vi "Get MAX rel move.vi"(0 "Zaber":T1={"Serial port handle"="", "Axis"="", "Controller #"=0, "Min position"=0.0, "Max position"=0.0, "Min velocity"=0.0, "Max velocity"=0.0, "Firmware"="", "Device ID"=0, "Variable event"=refnum, "Variable ref"=refnum, "Resolution, usteps/step"=0, "Serial port semaphore"=refnum, "Joystick buttons"={"MinDir"=1, "MaxDir"=2, "MedSpeed"=5, "HighSpeed"=6}} {"Joystick buttons"."HighSpeed" min=1 max=25 step=1; "Joystick buttons"."MedSpeed" min=1 max=25 step=1; "Joystick buttons"."MaxDir" min=1 max=25 step=1; "Joystick buttons"."MinDir" min=1 max=25 step=1}, 5 "error in":errorcluster) -> (14 "Zaber out":T1={"Serial port handle"="", "Axis"="", "Controller #"=0, "Min position"=0.0, "Max position"=0.0, "Min velocity"=0.0, "Max velocity"=0.0, "Firmware"="", "Device ID"=0, "Variable event"=refnum, "Variable ref"=refnum, "Resolution, usteps/step"=0, "Serial port semaphore"=refnum, "Joystick buttons"={"MinDir"=1, "MaxDir"=2, "MedSpeed"=5, "HighSpeed"=6}} {"Joystick buttons"."HighSpeed" min=1 max=25 step=1; "Joystick buttons"."MedSpeed" min=1 max=25 step=1; "Joystick buttons"."MaxDir" min=1 max=25 step=1; "Joystick buttons"."MinDir" min=1 max=25 step=1}, 16 "MAX rel move, usteps":i32, 19 "error out":errorcluster)   [LabVIEW 2017]
uses:
  CommandZaber.ctl
  GenericDataEvent/GenericEvent.ctl
  Zaber.ctl
  ZaberVariables.ctl
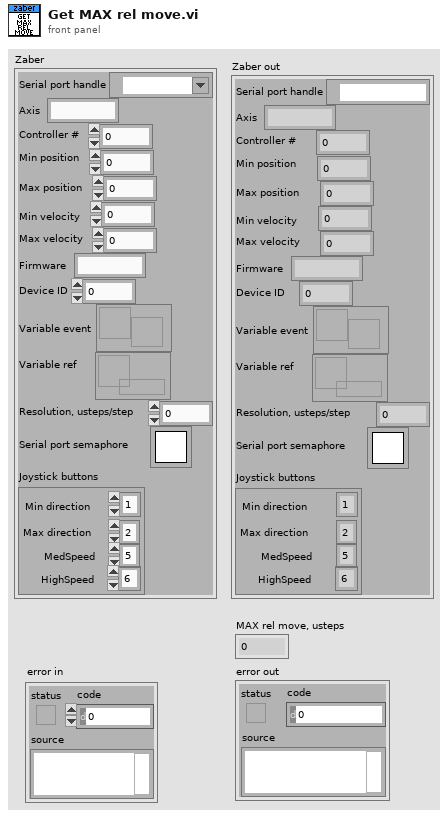
[diagram p1: front panel]
types:
  T1 = typedef "Zaber.ctl" = cluster{"Serial port handle":refnum<visa-resource-name>, "Axis":string, "Controller #":u8, "Min position":dbl, "Max position":dbl, "Min velocity":dbl, "Max velocity":dbl, "Firmware":string, "Device ID":i32, "Variable event":T2, "Variable ref":refnum<data-value>, "Resolution, usteps/step":i32, "Serial port semaphore":T3, "Joystick buttons":cluster{"MinDir":i32, "MaxDir":i32, "MedSpeed":i32, "HighSpeed":i32}}
  T2 = typedef "GenericEvent.ctl" = refnum<user-event>
  T3 = typedef "Semaphore RefNum" = refnum<k1>
  T4 = typedef "CommandZaber.ctl" = cluster{"Command":u8, "Data":i32}
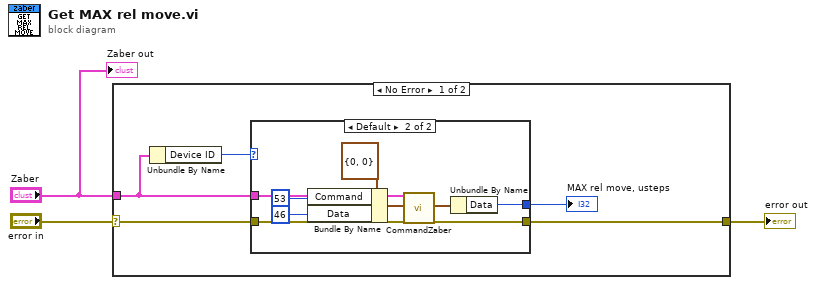
[diagram p0: block diagram]
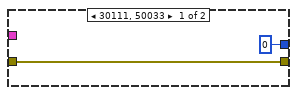
[diagram p2: hidden frame]
diagram:
  n1 = case shown="No Error" "error in" {
    selector: "error in" -> [w7 w20]
    tunnel: [w6 w20] -> w2
    tunnel: "Zaber" -> [w5 _]
    frame No Error {
      n2 = Unbundle By Name(w5) -> ("Device ID"=w4:i32)
      n3 = case shown="Default" w4 {
        tunnel: [0 ("Data") w19] -> w8
        tunnel: w7 -> [w10 w14]
        tunnel: [w10 w13] -> w6
        tunnel: w5 -> [_ w11]
        frame 30111, 50033 {
        }
        frame Default {
          n4 = Bundle By Name(cluster=T4 {"Command"=0, "Data"=0} ("Command"), "Command"=53 ("Data"), "Data"=46) -> (w17:T4)
          n5 = call "CommandZaber.vi"("Zaber"=w11, "Command"=w17, "error in"=w14) -> ("Answer"=w12:T4, "error out"=w13:errorcluster)  [unwired: 13 in, 2 out]
          n6 = Unbundle By Name(w12) -> ("Data"=w19:i32)
        }
      }
      "MAX rel move, usteps" <- w8
    }
    frame Error {
    }
  }
  "error out" <- w2
  "Zaber out" <- "Zaber"
